vi "Calculate Flatness.vi"(2 "Min Value":dbl, 3 "Max Value":dbl) -> (0 "Flatness":dbl)   [LabVIEW 2018, in "RDLUtilities.lvlib"]
uses:
  RDLUtilities.lvlib
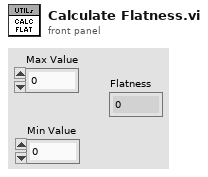
[diagram p1: front panel]
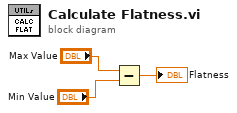
[diagram p0: block diagram]
diagram:
  n1 = Subtract(x="Max Value", y="Min Value") -> (x-y=→"Flatness":dbl)
